vi "check_has_tour_been_found.vi"(1 "no. of squares on chessboard":u8, 2 "tour in progress":T1[](array[typedef])) -> (0 "T = complete tour was found":bool)   [LabVIEW 2020, in "core.lvlib"]
uses:
  core.lvlib
  core_data/chessboard_index.ctl
  core_data/core_data.lvlib
panel:
  # "Development\ncontrols/indicators useful for development and testing, but which are not outputs of the VI"
  # "Input\nInputs to the VI"
  # "Output\nOutputs of the VI"
  # "Description\n\nBlank VI with error handling case. \n\nSummarize the use of this VI in this space."
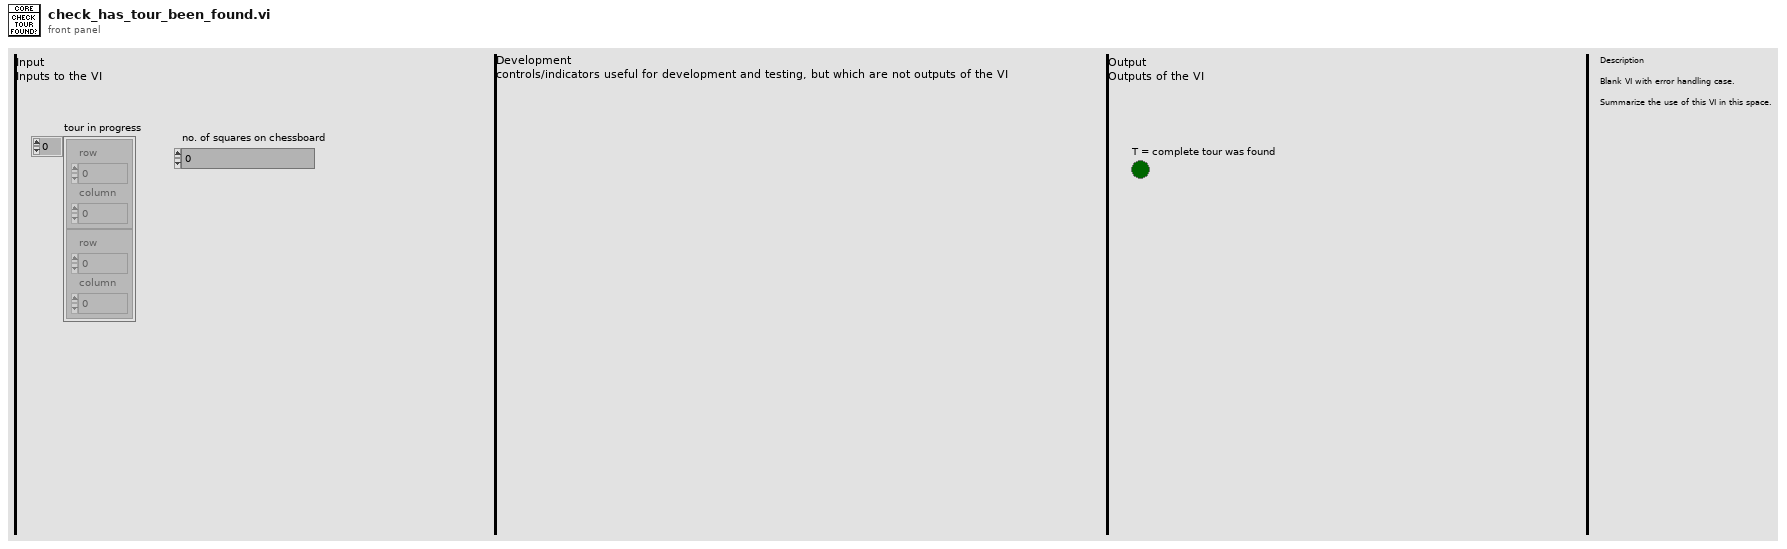
[diagram p1: front panel]
types:
  T1 = typedef "core.lvlib/core_data.lvlib/chessboard_index.ctl" = cluster{"row":u8, "column":u8}
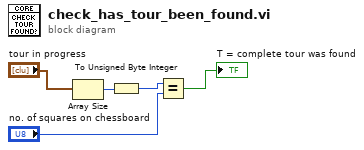
[diagram p0: block diagram]
diagram:
  n1 = Array Size(array="tour in progress") -> (size(s)=w4:i32)
  n2 = To Unsigned Byte Integer(number=w4) -> (unsigned 8bit integer=w3:u8)
  n3 = Equal?(x=w3, y="no. of squares on chessboard") -> (x = y?=→"T = complete tour was found":bool)
